vi "DisplaySequenceFile Event Callback.vi"(4 "GUI.lvlib:Auto UI.lvlib:Auto UI.lvclass":refnum<class "Auto UI.lvclass">, 5 "Event data":cluster{"file":refnum<k7>, "reason":i32}, 6 "CtlRef":refnum<k7>, 7 "Event common data":cluster{"Source":i32, "Type":u32, "Time":u32}) -> ()   [LabVIEW 2023, in "GUI.lvlib" / "Auto UI.lvlib" / "Auto UI.lvclass"]
uses:
  Auto UI.lvclass
  Auto UI.lvclass/Auto UI.ctl
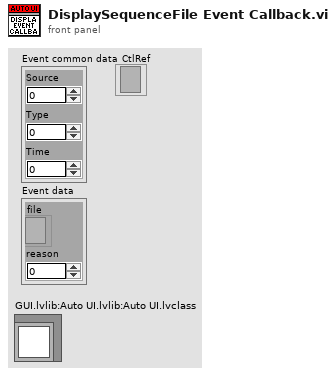
[diagram p1: front panel]
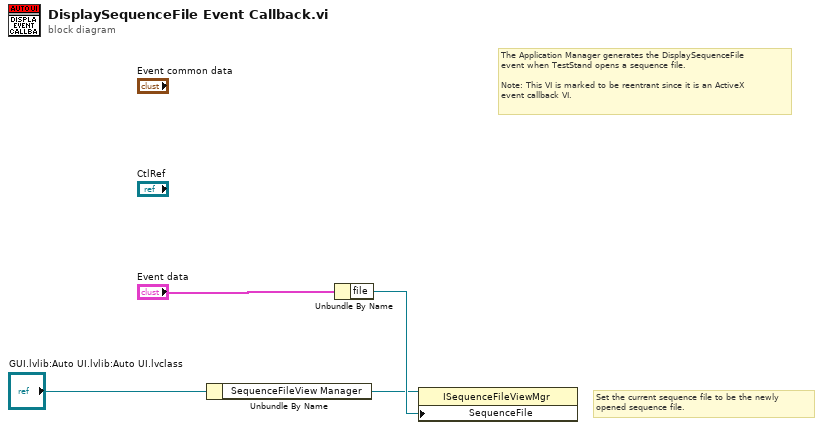
[diagram p0: block diagram]
diagram:
  # "Set the current sequence file to be the newly\nopened sequence file."
  # "The Application Manager generates the DisplaySequenceFile\nevent when TestStand opens a sequence file.\n\nNote: This VI is marked to be reentrant since it is an ActiveX\nevent callback VI."
  n1 = Unbundle By Name("GUI.lvlib:Auto UI.lvlib:Auto UI.lvclass") -> ("SequenceFileView Manager"=w2:refnum<k7>)
  n2 = Unbundle By Name("Event data") -> ("file"=w4:refnum<k7>)
  n3 = property class="ISequenceFileViewMgr"(reference=w2, "SequenceFile"=w4) -> ()  [unwired: 1 in, 2 out]
